vi "NO_CAM_Adjust Dashboard Window_NO_RESIZE.vi"(6 "Sizing Refnums":T1, 9 "Size Constraints":cluster{"min tab width":i32, "w/h":dbl}, 10 "VI":refnum<vi>, 11 "WIn Mode":refnum<notifier>) -> ()   [LabVIEW 2025]
panel:
  in  "Str Refnum":refnum<vi>
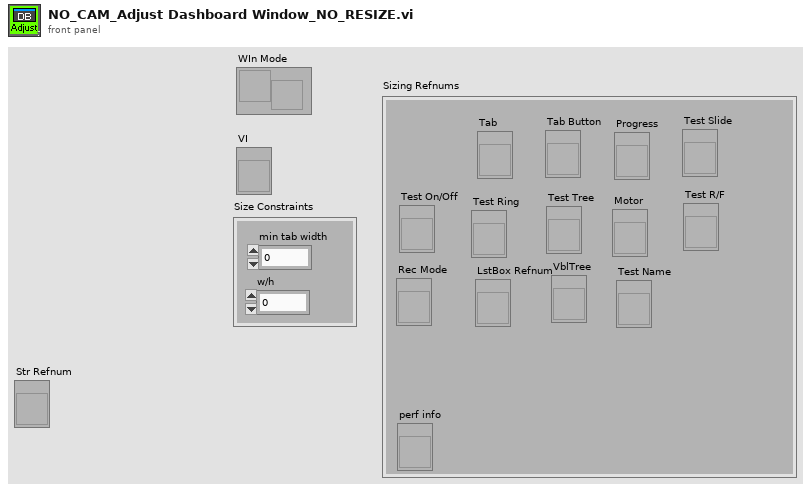
[diagram p1: front panel]
types:
  T1 = cluster{"Tab":refnum<vi>, "Tab Button":refnum<vi>, "Rec Mode":refnum<vi>, "Test Slide":refnum<vi>, "Test On/Off":refnum<vi>, "Test Ring":refnum<vi>, "Test R/F":refnum<vi>, "Test Name":refnum<vi>, "Motor":refnum<vi>, "Progress":refnum<vi>, "LstBox Refnum":refnum<vi>, "Test Tree":refnum<vi>, "VblTree":refnum<vi>, "perf info":refnum<vi>}
  T2 = typedef "LVRectTypeDef.ctl" = cluster{"Left":i16, "Top":i16, "Right":i16, "Bottom":i16}
  T3 = typedef "LVPointTypeDef.ctl" = cluster{"Horizontal":i16, "Vertical":i16}
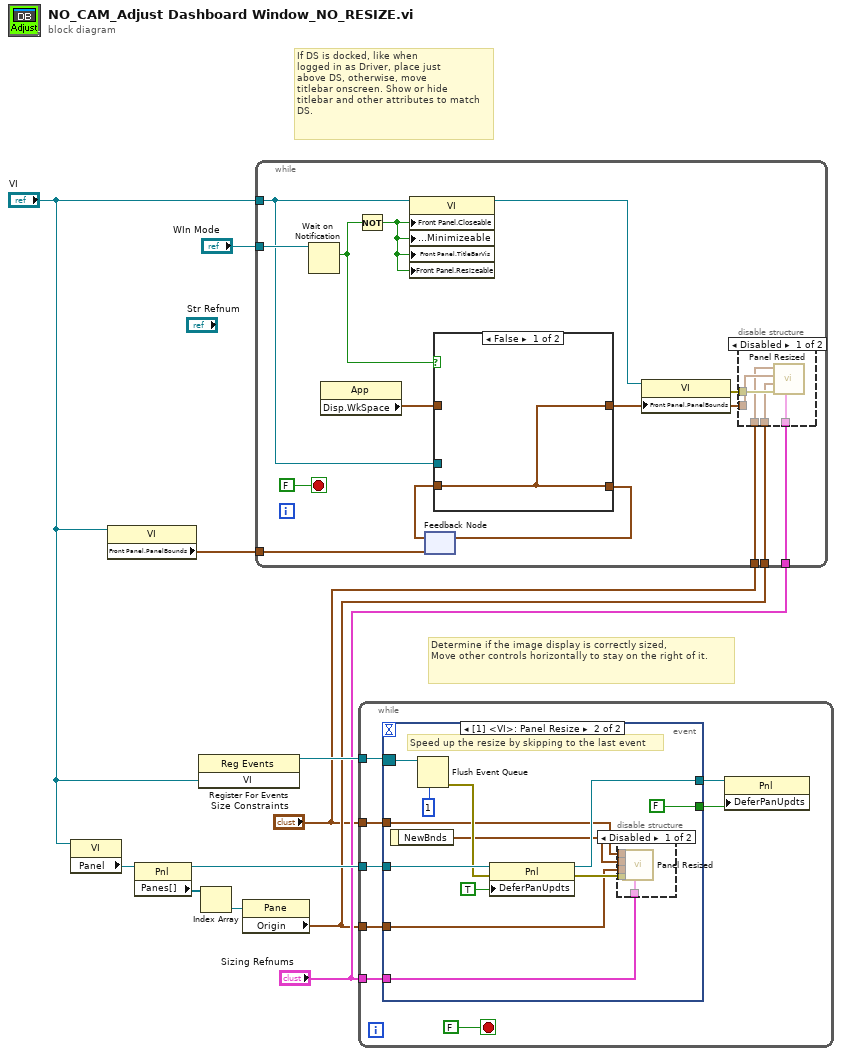
[diagram p0: block diagram]
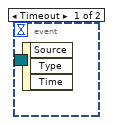
[diagram p2: hidden frame]
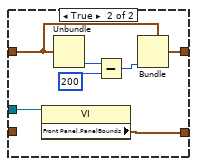
[diagram p5: hidden frame]
diagram:
  # "Determine if the image display is correctly sized,\nMove other controls horizontally to stay on the right of it."
  # "If DS is docked, like when\nlogged in as Driver, place just\nabove DS, otherwise, move\ntitlebar onscreen. Show or hide\ntitlebar and other attributes to match\nDS."
  n1 = property class="VI"(reference="VI") -> ("Panel"=w9:refnum<vi>)  [unwired: 1 in, 2 out]
  n2 = property class="VI"(reference="VI") -> ("Front Panel.PanelBounds"=w2:T2)  [unwired: 1 in, 2 out]
  n3 = property class="Pnl"(reference=w9) -> (reference out=w6:refnum<vi>, "Panes[]"=w8:refnum<vi>[])  [unwired: 1 in, 1 out]
  n4 = register-events("VI") -> (reference out=w10:refnum<event-registration>)  [unwired: 2 in, 1 out]
  n5 = Index Array(array=w8) -> (element=w7:refnum<vi>)  [unwired: 1 in]
  n6 = property class="Pane"(reference=w7) -> ("Origin"=w4:T3)  [unwired: 1 in, 2 out]
  n7 = while {
    tunnel: "WIn Mode" -> [w25]
    tunnel: "VI" -> [w16]
    tunnel: "Sizing Refnums" -> [w21]
    tunnel: w4 -> [w20]
    tunnel: "Size Constraints" -> [w18]
    tunnel: w2 -> [w13]
    stop <- FALSE stop-if-true
    n8 = Wait on Notification(notifier=w25) -> (notification=w17:bool)  [unwired: 3 in, 3 out]
    n9 = property class="App"() -> ("Disp.WkSpace"=w24:T2)  [unwired: 2 in, 2 out]
    n10 = Not(x=w17) -> (.not. x?=w12:bool)
    n11 = property class="VI"(reference=w16, "Front Panel.Closeable"=w12, "Front Panel.Minimizeable"=w12, "Front Panel.TitleBarVis"=w12, "Front Panel.Resizeable"=w12) -> (reference out=w23:refnum<vi>)  [unwired: 1 in, 1 out]
    n12 = feedback #1(w13) -> (w14:T2)
    n13 = case shown="False" w17 {
      tunnel: w24 -> [_ w35]
      tunnel: [w32 w36] -> w19
      tunnel: w16 -> [_ w34]
      tunnel: [w32 w33] -> w15
      tunnel: w14 -> [w32 _]
      frame False {
      }
      frame True {
        n14 = property class="VI"(reference=w34) -> ("Front Panel.PanelBounds"=w33:T2)  [unwired: 1 in, 2 out]
        n15 = Unbundle(w35) -> ("Bottom"=w39:i16)  [unwired: 3 out]
        n16 = Subtract(x=w39, y=200) -> (x-y=w37:i32)
        n17 = Bundle(cluster=w35, "Bottom"=w37) -> (w36:T2)  [unwired: 3 out]
      }
    }
    n18 = feedback-in #1(w15) -> ()
    n19 = property class="VI"(reference=w23, "Front Panel.PanelBounds"=w19) -> (error out=w22:errorcluster)  [unwired: 1 in, 1 out]
    n20 = disable-structure shown="Disabled" {
      disable-tunnel: w22 -> [w31 _]
      disable-tunnel: w21 -> [w30 _]
      disable-tunnel: w20 -> [w29 _]
      disable-tunnel: w19 -> [w28 _]
      disable-tunnel: w18 -> [w27 _]
      frame Disabled {
        n21 = call "Panel Resized.vi"("Sizing Refnums"=w30, "error in (no error)"=w31, "Origin"=w29, "NewBnds"=w28, "Size Constraints"=w27) -> ()  [unwired: 6 in, 1 out]
      }
      frame Enabled {
      }
    }
  }
  n22 = while {
    tunnel: w10 -> [w46]
    tunnel: "Sizing Refnums" -> [w45]
    tunnel: "Size Constraints" -> [w44]
    tunnel: w4 -> [w43]
    tunnel: w6 -> [w42]
    stop <- FALSE stop-if-true
    n23 = event shown="[1] <VI>: Panel Resize" {
      selector: w46 -> [_ w56]
      dyn-events: _ -> [_ _]
      timeout: _ -> [_ _]
      tunnel: w45 -> [_ w48]
      tunnel: w44 -> [_ w51]
      tunnel: w43 -> [_ w49]
      tunnel: w42 -> [_ w59]
      tunnel: [_ FALSE ("Defer Panel Updates")] -> w41
      tunnel: [_ w53] -> w40
      event Timeout {
        n24 = event-data() -> ()  [unwired: 1 in, 3 out]
      }
      event Panel Resize {
        # "Speed up the resize by skipping to the last event"
        n25 = event-data() -> ("NewBnds"=w50:T2)  [unwired: 1 in]
        n26 = Flush Event Queue(0:w56, 5:1 ("keep most recent")) -> (11:w54:errorcluster)  [unwired: 4 in, 2 out]
        n27 = property class="Pnl"(reference=w59, error in=w54, "DeferPanUpdts"=TRUE ("Defer Panel Updates")) -> (reference out=w53:refnum<vi>, error out=w52:errorcluster)
        n28 = disable-structure shown="Disabled" {
          disable-tunnel: w52 -> [w64 _]
          disable-tunnel: w51 -> [w63 _]
          disable-tunnel: w50 -> [w62 _]
          disable-tunnel: w49 -> [w61 _]
          disable-tunnel: w48 -> [w60 _]
          frame Disabled {
            n29 = call "Panel Resized.vi"("Sizing Refnums"=w60, "error in (no error)"=w64, "Origin"=w61, "NewBnds"=w62, "Size Constraints"=w63) -> ()  [unwired: 6 in, 1 out]
          }
          frame Enabled {
          }
        }
      }
    }
    n30 = property class="Pnl"(reference=w40, "DeferPanUpdts"=w41) -> ()  [unwired: 1 in, 2 out]
  }
